vi "Write Alias.vi"(8 "error in (no error)":errorcluster, 10 "Alias":string, 11 "Digital Multimeter in":refnum<class "Digital Multimeter.lvclass">) -> (0 "error out":errorcluster, 3 "Digital Multimeter out":refnum<class "Digital Multimeter.lvclass">)   [LabVIEW 2020, in "Digital Multimeter.lvclass"]
uses:
  Digital Multimeter.lvclass
  Digital Multimeter.lvclass/Digital Multimeter.ctl
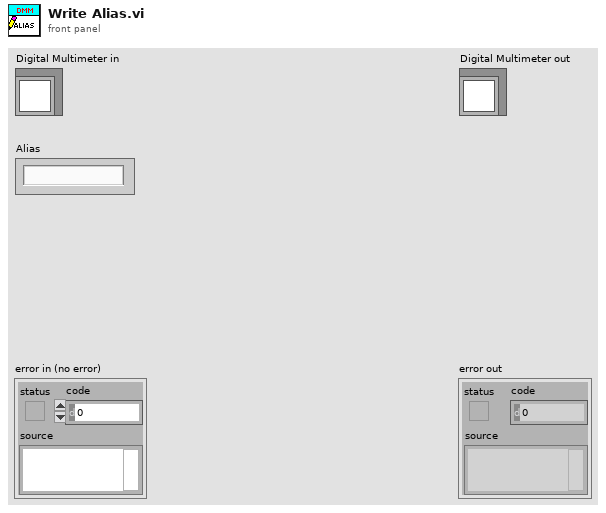
[diagram p1: front panel]
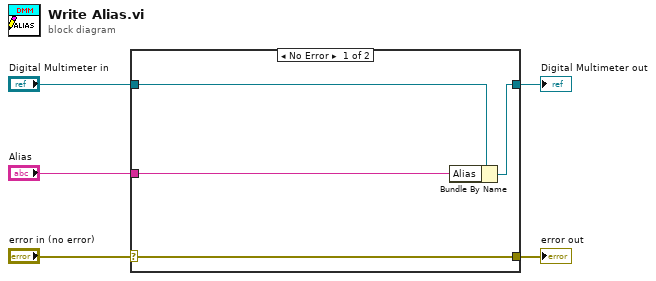
[diagram p0: block diagram]
diagram:
  n1 = case shown="No Error" "error in (no error)" {
    selector: "error in (no error)" -> [w9 w10]
    tunnel: [w9 w10] -> w4
    tunnel: [w7 w11] -> w2
    tunnel: "Digital Multimeter in" -> [w8 w11]
    tunnel: "Alias" -> [w6 _]
    frame No Error {
      n2 = Bundle By Name(cluster=w8, "Alias"=w6) -> (w7:refnum<class "Digital Multimeter.lvclass">)
    }
    frame Error {
    }
  }
  "error out" <- w4
  "Digital Multimeter out" <- w2
